vi "DrawLine3D_MultiColor.vi"(9 "Display":T1={"Mode"=enum."Inherit Value", "PointSize"=1.0, "LineWidth"=1.0}, 10 "Colors":u32[](array[colorbox]), 11 "Lines":cluster{"P0":T2, "P1":T2}[](array[cluster])) -> ()   [LabVIEW 2014]
uses:
  TypeDefs/Point3D.ctl
  <vilib>/picture/3D Picture Control/Object/Create Object (name).vi
  <vilib>/picture/3D Picture Control/Object/Add Object (no reference).vi
  <vilib>/picture/3D Picture Control/NI_3D Picture Control.lvlib
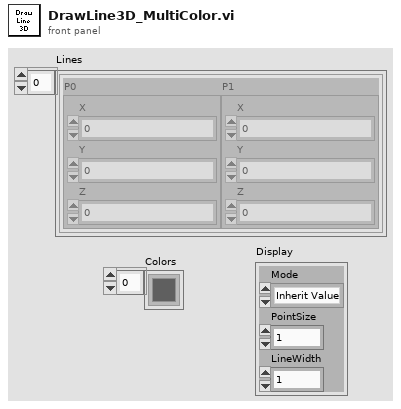
[diagram p1: front panel]
types:
  T1 = cluster{"Mode":enum16{"Inherit Value", "Points", "Wireframe", "Polygons"}, "PointSize":sgl, "LineWidth":sgl}
  T2 = typedef "Point3D.ctl" = cluster{"X":sgl, "Y":sgl, "Z":sgl}
  T3 = enum16{"Overall", "Per Primitive", "Per Vertex", "Binding Off"}
  T4 = enum16{"Points", "Lines", "Line Strip", "Line Loop", "Triangles", "Triangle Strip", "Triangle Fan", "Quads", "Quad Strip", "Polygon"}
  T5 = enum16{"New", "Find", "FindPattern", "GetTable", "Clear"}
  T6 = enum16{"Inherit Value", "Points", "Wireframe", "Polygons"}
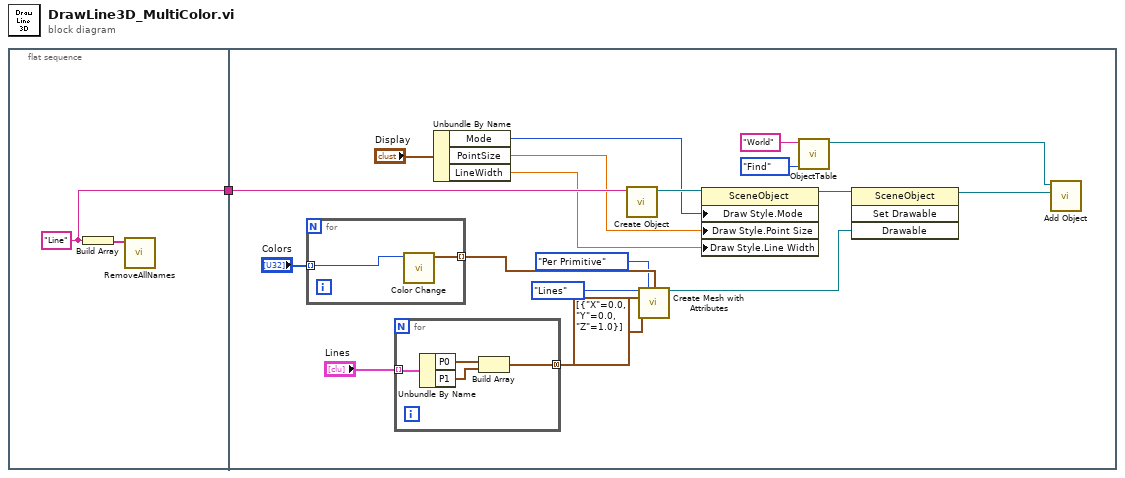
[diagram p0: block diagram]
diagram:
  n1 = flat-sequence {
    tunnel: [w2] -> w1
    tunnel: w1 -> [w12]
    frame #0 {
      w2 = "Line" ("string")
      n2 = Build Array(w2) -> (w3:string[])
      n3 = call "RemoveAllNames.vi"("Names"=w3) -> ()  [unwired: 11 in]
    }
    frame #1 {
      n4 = for {
        tunnel: [w24] -> w6 mode=indexing
        tunnel: "Colors" -> [w23] mode=indexing
        n5 = call <vilib>:"Color Change.vi"("Color"=w23) -> ("RGBA"=w24:cluster{"R":sgl, "G":sgl, "B":sgl, "A":sgl})  [unwired: 10 in]
      }
      n6 = for {
        tunnel: "Lines" -> [w28] mode=indexing
        tunnel: [w25] -> w15 mode=concatenating
        n7 = Unbundle By Name(w28) -> ("P0"=w27:T2, "P1"=w26:T2)
        n8 = Build Array(w27, w26) -> (w25:T2[])
      }
      n9 = Unbundle By Name("Display") -> ("Mode"=w10:T6, "PointSize"=w9:sgl, "LineWidth"=w8:sgl)
      n10 = call-poly <vilib>:"Create Object.vi"("Name"=w12) -> ("Scene:New Object"=w14:refnum<vi>)  [unwired: 9 in, 1 out]
      n11 = call <vilib>:"Create Mesh with Attributes.vi"("Draw Mode"=T4."Lines", "Color Binding Mode"=T3."Per Primitive", "Color Array"=w6, "Vertex Array"=w15, "Normal Array"=cluster{"X":sgl, "Y":sgl, "Z":sgl}[] [{"X"=0.0, "Y"=0.0, "Z"=1.0}]) -> ("New Mesh Refnum"=w17:refnum<vi>)  [unwired: 9 in, 1 out]
      n12 = property class="SceneObject"(reference=w14, "Draw Style.Mode"=w10, "Draw Style.Point Size"=w9, "Draw Style.Line Width"=w8) -> (reference out=w13:refnum<vi>)  [unwired: 1 in, 1 out]
      n13 = call "ObjectTable.vi"("ObjectStoreSelector"=T5."Find", "Name"="World") -> ("ObjectRef"=w18:refnum<vi>)  [unwired: 5 in, 4 out]
      n14 = invoke class="SceneObject" method="Set Drawable"(reference=w13, "Drawable"=w17) -> (reference out=w20:refnum<vi>)  [unwired: 2 in, 3 out]
      n15 = call-poly <vilib>:"Add Object.vi"("New Object In"=w20, "Scene Object In"=w18) -> ()  [unwired: 8 in, 2 out]
    }
  }
